vi "SCCAPI Get StaticVI Path.vi"(8 "error in (no error)":errorcluster, 10 "provider location":string) -> (0 "error out":errorcluster, 3 "staticVI path":path)   [LabVIEW 2017, in "NI_SCC.lvlib"]
uses:
  <vilib>/SourceControl/sccapi/NI_SCC.lvlib
  <vilib>/SourceControl/sccapi/SCCAPI SCC Operations.ctl
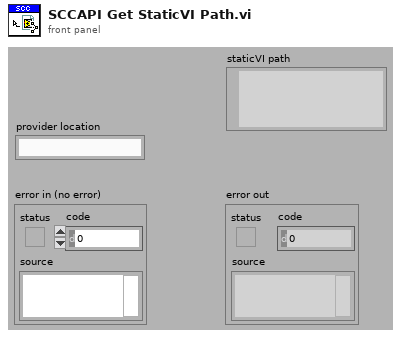
[diagram p1: front panel]
types:
  T1 = typedef "NI_SCC.lvlib/SCCAPI SCC Operations.ctl" = enum16{"Add", "Check In", "Check Out", "Close Project", "Compare Files", "Compare VIs", "Configure Project", "File History", "File Properties", "File Status", "Find All Providers", "Get Advanced Command Options", "Get File Copy", "Get Latest Version", "Get Project Name", "Get StaticVI Path", "Initialize", "Not A Source Control Reference", "Open Project", "Provider Supports Functionality", "Remove", "Run Provider", "Undo Check Out", "Uninitialize", "Is File In Local Path"}
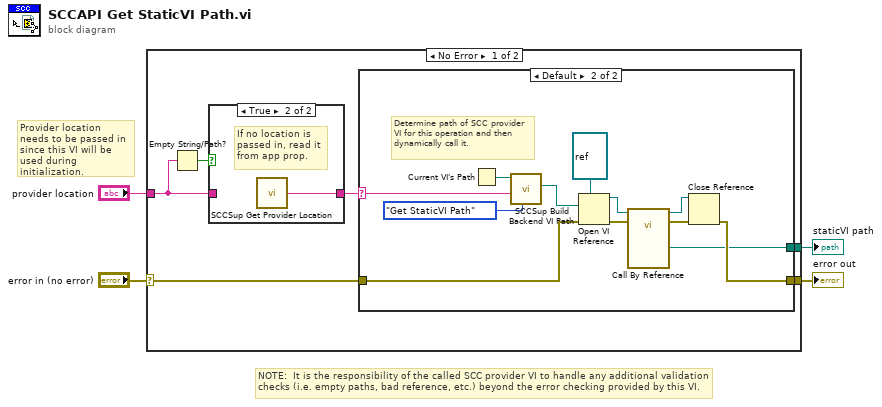
[diagram p0: block diagram]
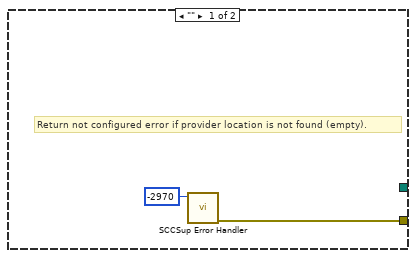
[diagram p3: hidden frame]
diagram:
  # "NOTE:  It is the responsibility of the called SCC provider VI to handle any additional validation checks (i.e. empty paths, bad reference, etc.) beyond the error checking provided by this VI."
  # "Provider location needs to be passed in  since this VI will be used during initialization."
  n1 = case shown="No Error" "error in (no error)" {
    selector: "error in (no error)" -> [w6 w27]
    tunnel: [w10 w27] -> w3
    tunnel: "provider location" -> [w8 _]
    tunnel: [w5 _] -> w1
    frame No Error {
      n2 = Empty String/Path?(string/path=w8) -> (empty?=w9:bool)
      n3 = case shown="True" w9 {
        tunnel: w8 -> [w11 _]
        tunnel: [w11 w12] -> w7
        frame False {
        }
        frame True {
          # "If no location is passed in, read it from app prop."
          n4 = call <vilib>:"SCCSup Get Provider Location.vi"() -> ("provider location"=w12:string)  [unwired: 6 in]
        }
      }
      n5 = case shown="Default" w7 {
        selector: w7 -> [_ w18]
        tunnel: [w13 w17] -> w10
        tunnel: w6 -> [_ w16]
        tunnel: [_ w15] -> w5
        frame "" {
          # "Return not configured error if provider location is not found (empty)."
          n6 = call <vilib>:"SCCSup Error Handler.vi"("scc error code"=-2970 ("code")) -> ("error out"=w13:errorcluster)  [unwired: 10 in]
        }
        frame Default {
          # "Determine path of SCC provider VI for this operation and then dynamically call it."
          n7 = Current VI's Path() -> (path=w21:path)
          n8 = call <vilib>:"SCCSup Build Backend VI Path.vi"("scc operation"=SCCAPI_SCC_Operations."Get StaticVI Path", "provider location"=w18, "caller path"=w21) -> ("scc backend VI path"=w20:path)  [unwired: 8 in]
          n9 = Open VI Reference(type specifier VI Refnum (for type only)=refnum<vi> refnum, vi path=w20, error in (no error)=w16) -> (vi reference=w25:refnum<vi>, error out=w24:errorcluster)  [unwired: 3 in]
          n10 = call-by-ref "?"(reference=w25, error in=w24) -> (reference out=w23:refnum<vi>, error out=w22:errorcluster, "staticVI path"=w15:path)  [unwired: 9 in]
          n11 = Close Reference(reference=w23, error in (no error)=w22) -> (error out=w17:errorcluster)
        }
      }
    }
    frame Error {
    }
  }
  "error out" <- w3
  "staticVI path" <- w1
